vi "Set Range.vi"(8 "Error In":errorcluster, 10 "Range":dbl, 11 "DMMIn":refnum<class "DMM.lvclass">) -> (0 "Error Out":errorcluster, 3 "DMMOut":refnum<class "DMM.lvclass">)   [LabVIEW 2019, in "DMM.lvclass"]
uses:
  DMM.lvclass
  DMM.lvclass/DMM.ctl
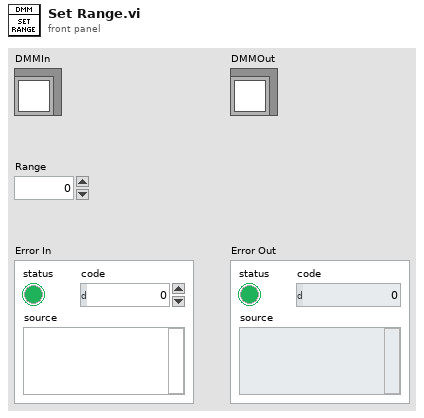
[diagram p1: front panel]
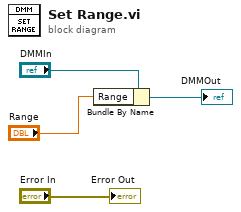
[diagram p0: block diagram]
diagram:
  n1 = Bundle By Name(cluster="DMMIn", "Range"="Range") -> (→"DMMOut":refnum<class "DMM.lvclass">)
  "Error Out" <- "Error In"
